vi "DriveExecuteCOPY.vi"(8 "error in (no error)":errorcluster) -> (0 "error out":errorcluster)   [LabVIEW 2023]
doc: "Execute for Drie\n\nClosed control loop for drive\n\ninput: \n error in (cluster)\n\noutput:\n error out (cluster)"
uses:
  <vilib>/Rock Robotics/WPI/ThirdParty/Phoenix-LabVIEW/Motor Controller/Controls/CTRE_Phoenix_MotorControl_ControlMode.ctl
  DriveGlobal.vi
  <vilib>/Rock Robotics/WPI/ThirdParty/JAS_Junk/TrajLib/Trajectory_Library.lvlib
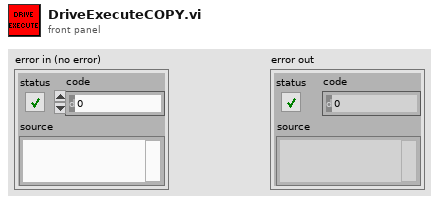
[diagram p1: front panel]
types:
  T1 = enum16{"Moving Average", "Low Pass 1st Order Butterworth", "Low Pass 2nd Order Butterworth", "High Pass 1st Order Butterworth", "High Pass 2nd Order Butterworth"}
  T2 = typedef "CTRE_Phoenix_MotorControl_ControlMode.ctl" = u16
  T3 = typedef "ADIS16470 Device Reference.ctl" = cluster{"DevStatus":errorcluster, "Hardware Config":T4, "Calibration Complete":refnum<notifier>, "Status Reference":refnum<data-value>, "Data Reference":refnum<data-value>, "Sychronous Process VI":T8, "Cmd FIFO":refnum<k33>, "Source":T9, "Data FIFO":refnum<k33>, "Calibration Time (ms)":u32, "Data Reference":refnum<data-value>}
  T4 = typedef "ADIS16470 Hardware Configuration.ctl" = cluster{"SPI Clock Rate (Hz)":dbl, "IMU SPI Mode (3)":T5, "IMU Reset Pin":T6, "IMU SPI Bus":T7, "IMU Data Ready Pin":T6, "Stall Config":cluster{"Pow2BytesPerRead":u8, "StallTicks":u16, "CsToSclkTicks":u8}}
  T5 = typedef "WPI_SPIMode.ctl" = enum16{"Mode 0 (Clk Idle Low,Sample on Leading)", "Mode 1 (Clk Idle Low,Sample on Trailing)", "Mode 2 (Clk Idle High,Sample on Leading)", "Mode 3 (Clk Idle High,Sample on Trailing)"}
  T6 = typedef "FPGA_DIOChannel.ctl" = enum8{"DIO 0", "DIO 1", "DIO 2", "DIO 3", "DIO 4", "DIO 5", "DIO 6", "DIO 7", "DIO 8", "DIO 9", "DIO MXP 0", "DIO MXP 1", "DIO MXP 2", "DIO MXP 3", "DIO MXP 4", "DIO MXP 5", "DIO MXP 6", "DIO MXP 7", "DIO MXP 8", "DIO MXP 9", "DIO MXP 10", "DIO MXP 11", "DIO MXP 12", "DIO MXP 13", "DIO MXP 14", "DIO MXP 15", "SPI Port CS1", "SPI Port CS2", "SPI Port CS3", "SPI Port MISO", "SPI Port MOSI", "Invalid"}
  T7 = typedef "spi_bus.ctl" = enum16{"SPI On-Board, CS0", "SPI On-Board, CS1", "SPI On-Board, CS2", "SPI On-Board, CS3", "SPI MXP", "Invalid"}
  T8 = typedef "ADIS16470 Process.ctl" = refnum<vi>
  T9 = typedef "FPGA_CounterEncoderSourceConvertionLVSourceType.ctl" = cluster{"DevStatus":errorcluster, "AnalogTriggerMode?":bool, "DigitalMode":cluster{"DIO Channel":T10}, "AnalogTriggerMode":cluster{"AnalogTriggerIndex":T11, "OutputType":T12}}
  T10 = typedef "FPGA_DIODigitalSourceChannel.ctl" = enum8{"DIO 0", "DIO 1", "DIO 2", "DIO 3", "DIO 4", "DIO 5", "DIO 6", "DIO 7", "DIO 8", "DIO 9", "DIO MXP 0", "DIO MXP 1", "DIO MXP 2", "DIO MXP 3", "DIO MXP 4", "DIO MXP 5", "DIO MXP 6", "DIO MXP 7", "DIO MXP 8", "DIO MXP 9", "DIO MXP 10", "DIO MXP 11", "DIO MXP 12", "DIO MXP 13", "DIO MXP 14", "DIO MXP 15", "SPI Port CS1", "SPI Port CS2", "SPI Port CS3", "SPI Port MISO", "SPI Port MOSI", "Disabled"}
  T11 = typedef "FPGA_AnalogTriggerIndex.ctl" = enum8{"Trig 0", "Trig 1", "Trig 2", "Trig 3", "Trig 4", "Trig 5", "Trig 6", "Trig 7", "Invalid"}
  T12 = typedef "FPGA_AnalogTriggerOutType.ctl" = enum16{"InWindow", "TriggerState", "Rising", "Falling"}
  T13 = typedef "ADIS16470 Status.ctl" = cluster{"Calibrated?":bool, "IMU Detected?":bool}
  T14 = typedef "ADIS16470 Data.ctl" = cluster{"XAngle":dbl, "YAngle":dbl, "ZAngle":dbl}
  T15 = typedef "Trajectory_Library.lvlib/SIMPLE_MOTOR_FF.ctl" = cluster{"Ks":dbl, "Kv":dbl, "Ka":dbl, "KnInv":dbl}
  T16 = typedef "Trajectory_Library.lvlib/PID_ADV_LIMITS.ctl" = cluster{"MaxInput":dbl, "MinInput":dbl, "Continuous":bool, "MaxOutput":dbl, "MinOutput":dbl}
  T17 = typedef "Trajectory_Library.lvlib/PID_ADV_TUNING.ctl" = cluster{"Kf":dbl, "Kp":dbl, "Ki":dbl, "Kd":dbl, "MaximumIntegral":dbl, "MinimumIntegral":dbl, "Filter Derivative":bool}
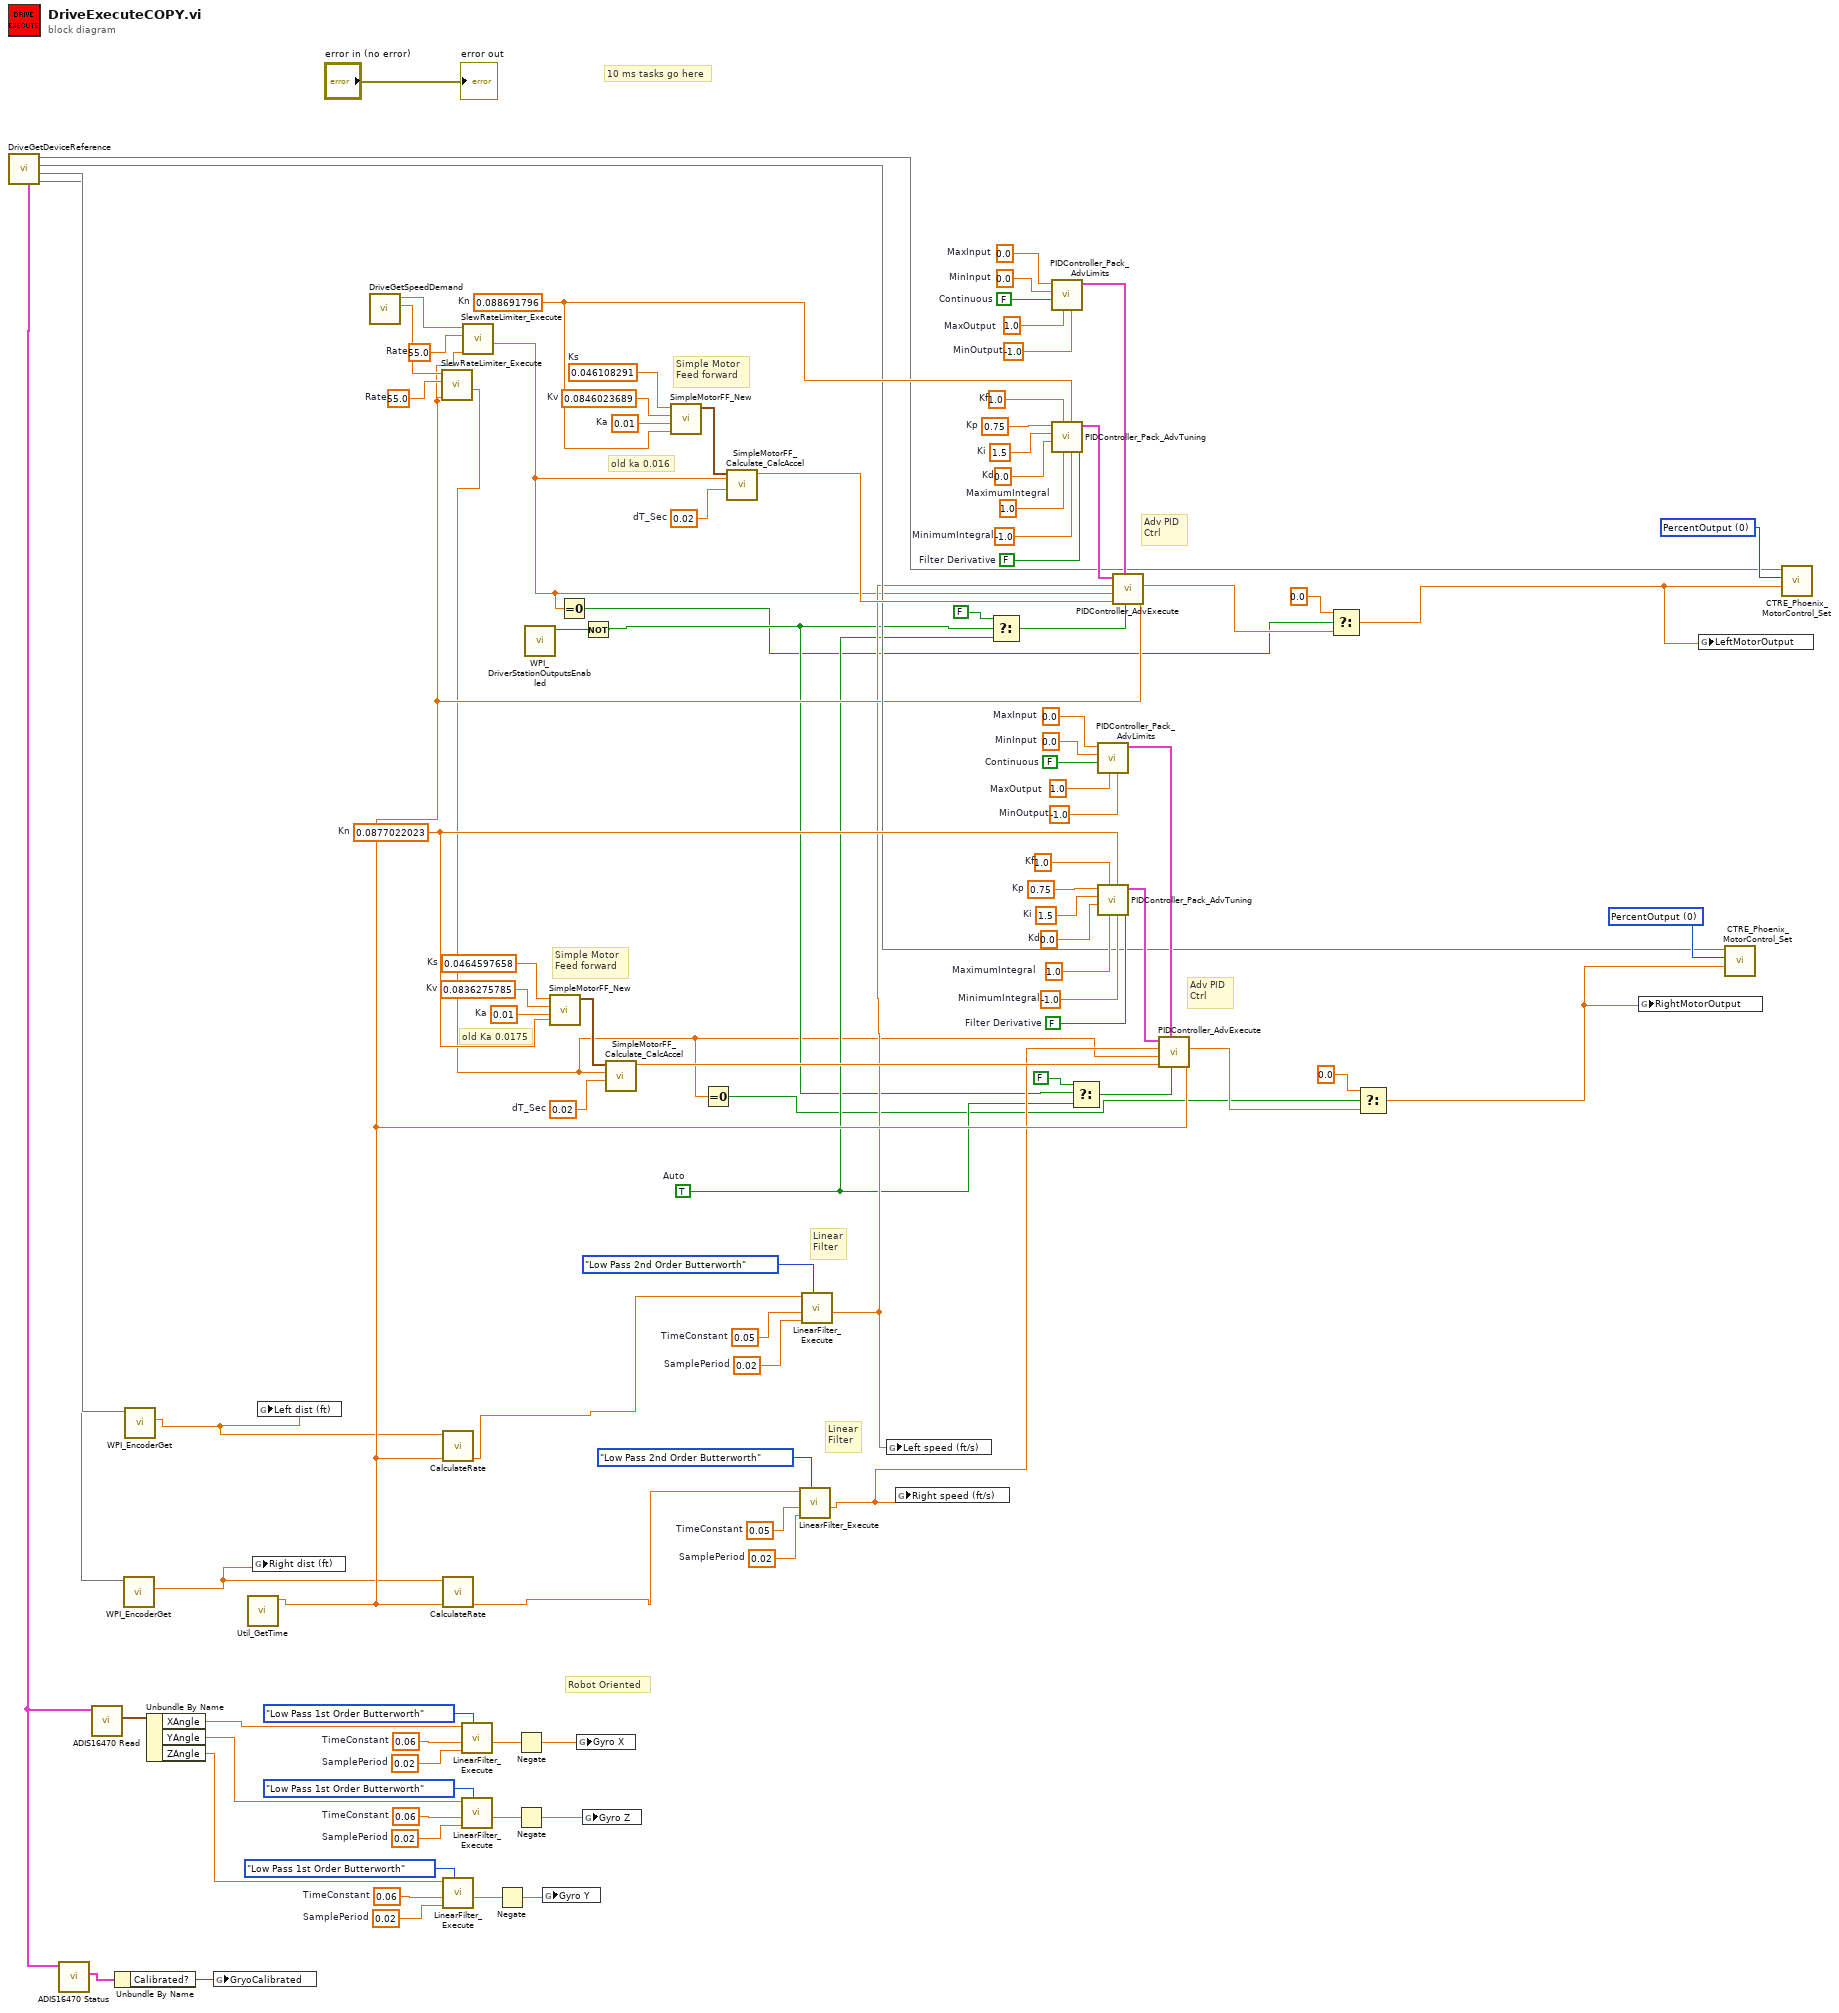
[diagram p0: block diagram]
diagram:
  w8 = 0.02  # SamplePeriod
  w7 = 0.06  # TimeConstant
  w14 = 0.02  # SamplePeriod
  w13 = 0.06  # TimeConstant
  w19 = 0.02  # SamplePeriod
  w18 = 0.06  # TimeConstant
  w47 = 0.02  # SamplePeriod
  w46 = 0.05  # TimeConstant
  w51 = 0.02  # SamplePeriod
  w50 = 0.05  # TimeConstant
  w56 = 55.0  # Rate
  w58 = 55.0  # Rate
  w33 = TRUE  # Auto
  w63 = 0.0877022023  # Kn
  w78 = 0.75  # Kp
  w77 = 1.5  # Ki
  w76 = 0.0  # Kd
  w75 = 1.0  # Kf
  w74 = 1.0  # MaximumIntegral
  w73 = -1.0  # MinimumIntegral
  w72 = FALSE  # Filter Derivative
  w70 = 0.0  # MinInput
  w69 = FALSE  # Continuous
  w68 = 1.0  # MaxOutput
  w71 = -1.0  # MinOutput
  w67 = 0.0  # MaxInput
  w64 = 0.088691796  # Kn
  w91 = 0.75  # Kp
  w53 = 1.5  # Ki
  w90 = 0.0  # Kd
  w89 = 1.0  # Kf
  w88 = 1.0  # MaximumIntegral
  w87 = -1.0  # MinimumIntegral
  w86 = FALSE  # Filter Derivative
  w84 = 0.0  # MinInput
  w83 = FALSE  # Continuous
  w82 = 1.0  # MaxOutput
  w85 = -1.0  # MinOutput
  w81 = 0.0  # MaxInput
  w96 = 0.02  # dT_Sec
  w94 = 0.0464597658  # Ks
  w93 = 0.0836275785  # Kv
  w92 = 0.01  # Ka
  w101 = 0.02  # dT_Sec
  w99 = 0.046108291  # Ks
  w98 = 0.0846023689  # Kv
  w97 = 0.01  # Ka
  w104 = T2 0 items=["PercentOutput"=0, "Position"=1, "Velocity"=2, "Current"=3, "Follower"=5, "MotionProfile"=6, "MotionMagic"=7, "MotionProfileArc"=10, "Disabled"=15] ("Control Mode")
  w105 = T2 0 items=["PercentOutput"=0, "Position"=1, "Velocity"=2, "Current"=3, "Follower"=5, "MotionProfile"=6, "MotionMagic"=7, "MotionProfileArc"=10, "Disabled"=15] ("Control Mode")
  # "Robot Oriented"
  # "old Ka 0.0175"
  # "old ka 0.016"
  # "Linear\nFilter"
  # "Linear\nFilter"
  # "Adv PID\nCtrl"
  # "Adv PID\nCtrl"
  # "Simple Motor\nFeed forward"
  # "Simple Motor\nFeed forward"
  # "10 ms tasks go here"
  n1 = call "DriveGetDeviceReference.vi"() -> (0:w28, 1:w29, 2:w59, 3:w60, "Gryo"=w30:T3)  [unwired: 7 in]
  n2 = call <vilib>:"ADIS16470 Status.vi"("ADIS16470DevRef"=w30) -> ("ADIS16470 Status"=w32:T13)  [unwired: 8 in, 2 out]
  n3 = call <vilib>:"ADIS16470 Read.vi"("ADIS16470DevRef"=w30) -> ("ADIS16470 Value"=w102:T14)  [unwired: 7 in, 3 out]
  n4 = Unbundle By Name(w32) -> ("Calibrated?"=w31:bool)
  n5 = call <vilib>:"WPI_EncoderGet.vi"("EncoderDevRef"=w28) -> ("Distance"=w27:dbl)  [unwired: 5 in, 5 out]
  n6 = call <vilib>:"WPI_EncoderGet.vi"("EncoderDevRef"=w29) -> ("Distance"=w26:dbl)  [unwired: 5 in, 5 out]
  n7 = Unbundle By Name(w102) -> ("XAngle"=w3:dbl, "YAngle"=w10:dbl, "ZAngle"=w16:dbl)
  n8 = global write "DriveGlobal.vi" "GryoCalibrated"(w31) -> ()
  n9 = call <vilib>:"Util_GetTime.vi"() -> ("FPGA_Time_Seconds"=w52:dbl)  [unwired: 9 in, 2 out]
  n10 = global write "DriveGlobal.vi" "Right dist (ft)"(w27) -> ()
  n11 = global write "DriveGlobal.vi" "Left dist (ft)"(w26) -> ()
  n12 = call "DriveGetSpeedDemand.vi"() -> ("vY"=w55:dbl, "vX"=w57:dbl)  [unwired: 8 in, 2 out]
  n13 = call <vilib>:"SlewRateLimiter_Execute.vi"("Time"=w52, "PositiveRate"=w56, "Input"=w55) -> ("Output"=w21:dbl)  [unwired: 7 in, 1 out]
  n14 = call "CalculateRate.vi"("Time (s)"=w52, "Distance (units)"=w26) -> ("Rate (units/s)"=w2:dbl)  [unwired: 9 in]
  n15 = call "CalculateRate.vi"("Time (s)"=w52, "Distance (units)"=w27) -> ("Rate (units/s)"=w1:dbl)  [unwired: 9 in]
  n16 = call <vilib>:"LinearFilter_Execute.vi"("Filter Type"=T1."Low Pass 1st Order Butterworth", "SamplePeriod"=w19, "TimeConstant"=w18, "Input"=w16) -> ("Output"=w15:dbl)  [unwired: 6 in, 1 out]
  n17 = call <vilib>:"LinearFilter_Execute.vi"("Filter Type"=T1."Low Pass 1st Order Butterworth", "SamplePeriod"=w8, "TimeConstant"=w7, "Input"=w3) -> ("Output"=w5:dbl)  [unwired: 6 in, 1 out]
  n18 = call <vilib>:"LinearFilter_Execute.vi"("Filter Type"=T1."Low Pass 1st Order Butterworth", "SamplePeriod"=w14, "TimeConstant"=w13, "Input"=w10) -> ("Output"=w11:dbl)  [unwired: 6 in, 1 out]
  n19 = call <vilib>:"SlewRateLimiter_Execute.vi"("Time"=w52, "PositiveRate"=w58, "Input"=w57) -> ("Output"=w23:dbl)  [unwired: 7 in, 1 out]
  n20 = Negate(x=w15) -> (-x=w54:dbl)
  n21 = Negate(x=w5) -> (-x=w4:dbl)
  n22 = Negate(x=w11) -> (-x=w9:dbl)
  n23 = call <vilib>:"WPI_DriverStationOutputsEnabled.vi"() -> ("OutputsEnabled?"=w25:bool)  [unwired: 10 in, 1 out]
  n24 = global write "DriveGlobal.vi" "Gyro Y"(w54) -> ()
  n25 = call <vilib>:"SimpleMotorFF_New.vi"("Kn"=w63, "Ka"=w92, "Kv"=w93, "Ks"=w94) -> ("SIMPLE_MOTOR_FF"=w95:T15)  [unwired: 7 in]
  n26 = Equal To 0?(x=w23) -> (x = 0?=w22:bool)
  n27 = global write "DriveGlobal.vi" "Gyro X"(w4) -> ()
  n28 = Not(x=w25) -> (.not. x?=w24:bool)
  n29 = global write "DriveGlobal.vi" "Gyro Z"(w9) -> ()
  n30 = call <vilib>:"SimpleMotorFF_Calculate_CalcAccel.vi"("dT_Sec"=w96, "VelSp"=w21, "SIMPLE_MOTOR_FF"=w95) -> ("FeedForward"=w61:dbl)  [unwired: 8 in]
  n31 = call <vilib>:"SimpleMotorFF_New.vi"("Kn"=w64, "Ka"=w97, "Kv"=w98, "Ks"=w99) -> ("SIMPLE_MOTOR_FF"=w100:T15)  [unwired: 7 in]
  n32 = Equal To 0?(x=w21) -> (x = 0?=w20:bool)
  n33 = call <vilib>:"SimpleMotorFF_Calculate_CalcAccel.vi"("dT_Sec"=w101, "VelSp"=w23, "SIMPLE_MOTOR_FF"=w100) -> ("FeedForward"=w62:dbl)  [unwired: 8 in]
  n34 = call <vilib>:"LinearFilter_Execute.vi"("Filter Type"=T1."Low Pass 2nd Order Butterworth", "SamplePeriod"=w47, "TimeConstant"=w46, "Input"=w1) -> ("Output"=w44:dbl)  [unwired: 6 in, 1 out]
  n35 = call <vilib>:"LinearFilter_Execute.vi"("Filter Type"=T1."Low Pass 2nd Order Butterworth", "SamplePeriod"=w51, "TimeConstant"=w50, "Input"=w2) -> ("Output"=w48:dbl)  [unwired: 6 in, 1 out]
  n36 = global write "DriveGlobal.vi" "Left speed (ft/s)"(w48) -> ()
  n37 = global write "DriveGlobal.vi" "Right speed (ft/s)"(w44) -> ()
  n38 = Select(t=FALSE, s=w24, f=w33) -> (s? t:f=w43:bool)
  n39 = call <vilib>:"PIDController_Pack_AdvLimits.vi"("MinOutput"=w85, "MaxOutput"=w82, "Continuous"=w83, "MinInput"=w84, "MaxInput"=w81) -> ("Adv PID Limits"=w79:T16)  [unwired: 6 in]
  n40 = call <vilib>:"PIDController_Pack_AdvTuning.vi"("Filter Derivative"=w86, "MinimumIntegral"=w87, "Kn"=w64, "MaximumIntegral"=w88, "Kf"=w89, "Kd"=w90, "Ki"=w53, "Kp"=w91) -> ("Adv PID Tuning"=w80:T17)  [unwired: 3 in]
  n41 = Select(t=FALSE, s=w24, f=w33) -> (s? t:f=w34:bool)
  n42 = call <vilib>:"PIDController_Pack_AdvLimits.vi"("MinOutput"=w71, "MaxOutput"=w68, "Continuous"=w69, "MinInput"=w70, "MaxInput"=w67) -> ("Adv PID Limits"=w65:T16)  [unwired: 6 in]
  n43 = call <vilib>:"PIDController_Pack_AdvTuning.vi"("Filter Derivative"=w72, "MinimumIntegral"=w73, "Kn"=w63, "MaximumIntegral"=w74, "Kf"=w75, "Kd"=w76, "Ki"=w77, "Kp"=w78) -> ("Adv PID Tuning"=w66:T17)  [unwired: 3 in]
  n44 = call <vilib>:"PIDController_AdvExecute.vi"("Time"=w52, "Auto"=w43, "Adv PID Limits"=w79, "FF-FeedForward"=w62, "SP-SetPoint"=w23, "PV-Measurement"=w48, "Adv PID Tuning"=w80) -> ("CO-ControlOutput"=w41:dbl)  [unwired: 2 in, 2 out]
  n45 = call <vilib>:"PIDController_AdvExecute.vi"("Time"=w52, "Auto"=w34, "Adv PID Limits"=w65, "FF-FeedForward"=w61, "SP-SetPoint"=w21, "PV-Measurement"=w44, "Adv PID Tuning"=w66) -> ("CO-ControlOutput"=w36:dbl)  [unwired: 2 in, 2 out]
  n46 = Select(t=0.0, s=w22, f=w41) -> (s? t:f=w40:dbl)
  n47 = Select(t=0.0, s=w20, f=w36) -> (s? t:f=w37:dbl)
  n48 = global write "DriveGlobal.vi" "RightMotorOutput"(w37) -> ()
  n49 = global write "DriveGlobal.vi" "LeftMotorOutput"(w40) -> ()
  n50 = call <vilib>:"CTRE_Phoenix_MotorControl_Set.vi"("Output"=w37, "Control Mode"=w104, "PhoenixMotorControlDevRef"=w59) -> ()  [unwired: 7 in, 2 out]
  n51 = call <vilib>:"CTRE_Phoenix_MotorControl_Set.vi"("Output"=w40, "Control Mode"=w105, "PhoenixMotorControlDevRef"=w60) -> ()  [unwired: 7 in, 2 out]
  "error out" <- "error in (no error)"
